vi "Start Target.vi"(7 "Target Ident":string, 8 "error in":errorcluster, 11 "Host Measure and Stimulus Subsystems in":refnum<class "Measure and Stimulus Subsystems.lvclass">) -> (0 "error out":errorcluster, 3 "Host Measure and Stimulus Subsystems out":refnum<class "Measure and Stimulus Subsystems.lvclass">)   [LabVIEW 2023, in "HAL GOOP4.lvlib" / "Measure and Stimulus Subsystems.lvclass"]
uses:
  Measure and Stimulus Subsystems.lvclass
  Measure and Stimulus Subsystems.lvclass/Measure and Stimulus Subsystems.ctl
  <vilib>/Utility/error.llb/Error Cluster From Error Code.vi
  <vilib>/ErrorRing/Error Ring.xnode
  Virt Instr Host/Virt Instr Host.lvclass
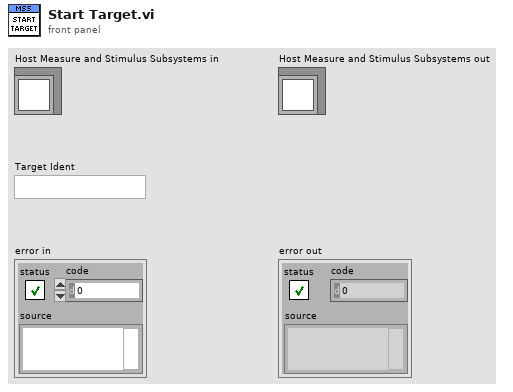
[diagram p1: front panel]
types:
  T1 = map{string, refnum<class "Virt Instr Host.lvclass">}
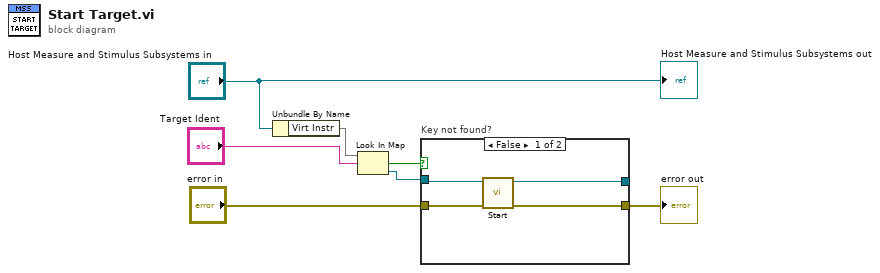
[diagram p0: block diagram]
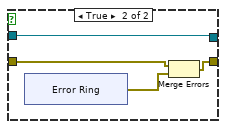
[diagram p2: hidden frame]
diagram:
  n1 = Unbundle By Name("Host Measure and Stimulus Subsystems in") -> ("Virt Instr"=w4:T1)
  n2 = Look In Map(map=w4, key="Target Ident") -> (key not found?=w1:bool, value=w3:refnum<class "Virt Instr Host.lvclass">)  [unwired: 1 in]
  n3 = case "Key not found?" shown="False" w1 {
    tunnel: w3 -> [w10 w12]
    tunnel: "error in" -> [w11 w13]
    tunnel: [w9 w12] -> _
    tunnel: [w8 w15] -> w6
    frame False {
      n4 = call-dynamic "Start.vi"("error in (no error)"=w11, "Virt Instr Base in"=w10) -> ("error out"=w8:errorcluster, "Virt Instr Base out"=w9:refnum<class "Virt Instr Host.lvclass">)  [unwired: 8 in]
    }
    frame True {
      n5 = xnode "Error Ring"() -> ("error out"=w14:errorcluster)
      n6 = Merge Errors(w13, w14) -> (w15:errorcluster)
    }
  }
  "error out" <- w6
  "Host Measure and Stimulus Subsystems out" <- "Host Measure and Stimulus Subsystems in"
